vi "OpenMV_SelectLab.vi"(2 "ROI":T1, 3 "image":picture) -> (0 "ROI out":T1, 1 "thresholds":dbl[](array[numeric])=[90.0, 10.0, 20.0, -20.0, 20.0, -20.0])   [LabVIEW 2020]
doc: "This VI pops up a window where the user can select a region of interest."
panel:
  out "Plots":T2
  out "Mouse Down":cluster{"X":i32, "Y":i32}
  out "String":string
  out "Mouse in":bool
  in  "Pen":u32(colorbox)=16774656
  out "overlay":picture caption="Image"
  in  "OK":bool
  out "Display":picture caption="new picture"
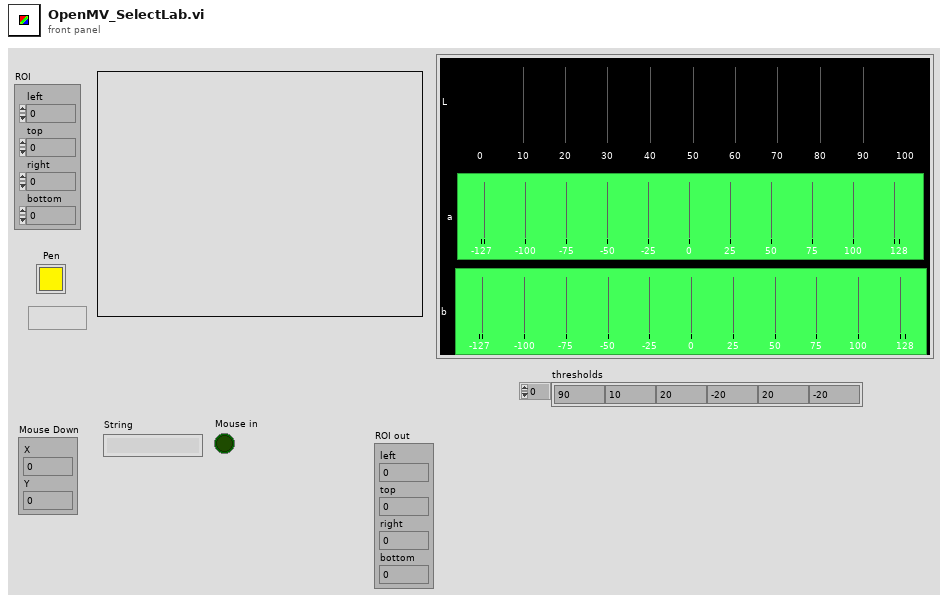
[diagram p1: front panel]
types:
  T1 = cluster{"left":i32, "top":i32, "right":i32, "bottom":i32}
  T2 = cluster{"L":dbl[], "a":cluster{i32, i32, dbl[]}, "b":cluster{i32, i32, dbl[]}}
  T3 = typedef "imagedata.ctl" = cluster{"image type":i32, "image depth":i32, "image":u8[], "mask":u8[], "colors":u32[], "Rectangle":cluster{"left":i16, "top":i16, "right":i16, "bottom":i16}}
  T4 = cluster{"left":i16, "top":i16, "right":i16, "bottom":i16}
  T5 = typedef "LVMouseTypeDef.ctl" = cluster{"Mouse Position":cluster{"X":i32, "Y":i32}, "Mouse Modifiers":cluster{"Button Down":bool, "Shift Mod":bool, "Menu Mod":bool, "Option Mod":bool}}
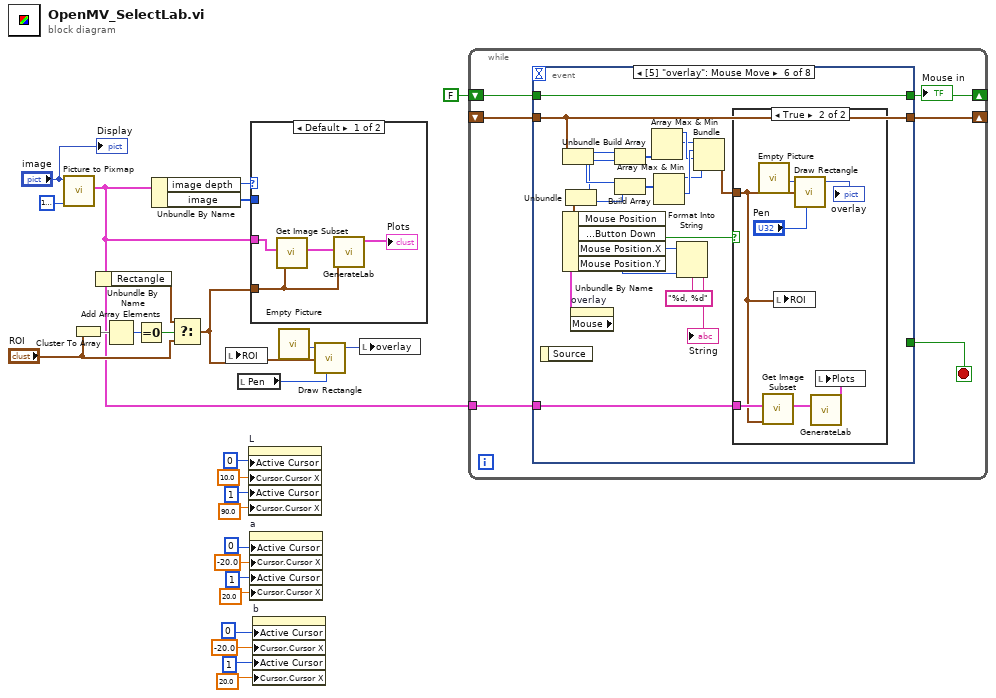
[diagram p0: block diagram]
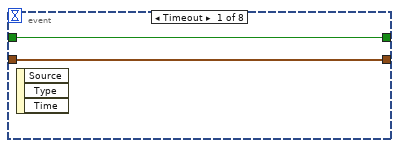
[diagram p3: hidden frame]
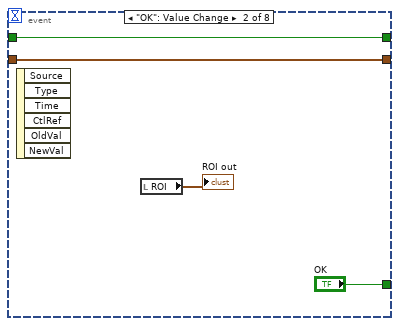
[diagram p4: hidden frame]
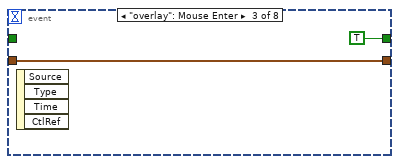
[diagram p5: hidden frame]
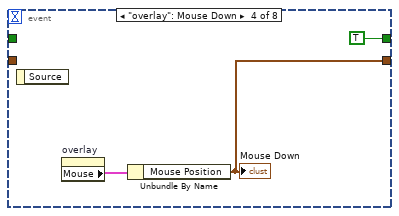
[diagram p6: hidden frame]
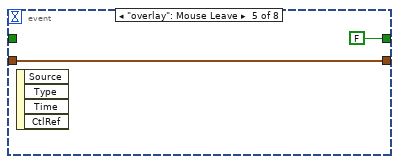
[diagram p7: hidden frame]
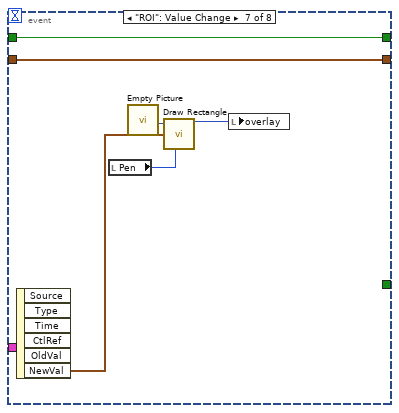
[diagram p9: hidden frame]
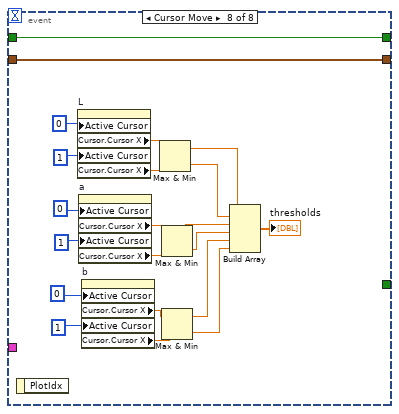
[diagram p10: hidden frame]
diagram:
  n1 = call <vilib>:"Picture to Pixmap.vi"("Background Color"=u32 16777216, "picture"="image") -> ("image data"=w2:T3)  [unwired: 8 in, 1 out]
  n2 = Cluster To Array(cluster="ROI") -> (array=w7:i32[])
  n3 = Unbundle By Name(w2) -> ("Rectangle"=w1:T4)
  n4 = Add Array Elements(numeric array=w7) -> (sum=w6:i32)
  n5 = Equal To 0?(x=w6) -> (x = 0?=w5:bool)
  n6 = Unbundle By Name(w2) -> ("image depth"=w25:i32, "image"=w24:u8[])
  n7 = Select(t=w1, s=w5, f="ROI") -> (s? t:f=w3:T1)
  n8 = local write "ROI"(w3) -> ()
  n9 = local read "Pen"() -> (w8:u32)
  n10 = property on="L" class="WFGraph (strict)"("Active Cursor"=u32 0, "Cursor.Cursor X"=10.0 ("Cursor.Cursor Position:Cursor X"), "Active Cursor"=u32 1, "Cursor.Cursor X"=90.0 ("Cursor.Cursor Position:Cursor X")) -> ()  [unwired: 2 in, 2 out]
  n11 = property on="a" class="WFGraph (strict)"("Active Cursor"=u32 0, "Cursor.Cursor X"=-20.0 ("Cursor.Cursor Position:Cursor X"), "Active Cursor"=u32 1, "Cursor.Cursor X"=20.0 ("Cursor.Cursor Position:Cursor X")) -> ()  [unwired: 2 in, 2 out]
  n12 = case shown="Default" w25 {
    tunnel: w24 -> [_ _]
    tunnel: w2 -> [w30 _]
    tunnel: w3 -> [w28 _]
    frame Default {
      n13 = call <vilib>:"Get Image Subset.vi"("subset rect"=w28, "image data"=w30) -> ("image subset"=w29:T3)  [unwired: 4 in, 1 out]
      n14 = call "GenerateLab.vi"("ROI"=w28, "image data"=w29) -> ("Plots"=→"Plots":T2)  [unwired: 8 in, 1 out]
    }
    frame ..8 {
    }
  }
  n15 = property on="b" class="WFGraph (strict)"("Active Cursor"=u32 0, "Cursor.Cursor X"=-20.0 ("Cursor.Cursor Position:Cursor X"), "Active Cursor"=u32 1, "Cursor.Cursor X"=20.0 ("Cursor.Cursor Position:Cursor X")) -> ()  [unwired: 2 in, 2 out]
  n16 = call "Empty Picture"() -> ("empty picture"=w10:picture)
  n17 = call <vilib>:"Draw Rectangle.vi"("picture"=w10, "rect"=w3, "color(black)"=w8) -> ("new picture"=w9:picture)  [unwired: 6 in]
  n18 = local write "overlay"(w9) -> ()
  n19 = while {
    shift-right: [w36] -> _
    shift-left: FALSE ("Mouse in") -> [w35]
    shift-right: [w34] -> _
    shift-left: _ -> [w33]
    tunnel: w2 -> [w32]
    stop <- w37 stop-if-true
    n20 = event shown="[5] \"overlay\": Mouse Move" {
      selector: _ -> [_ _ _ _ _ _ _ _]
      dyn-events: _ -> [_ _ _ _ _ _ _ _]
      timeout: _ -> [_ _ _ _ _ _ _ _]
      tunnel: [_ "OK" _ _ _ _ _ _] -> w37
      tunnel: [w39 w42 TRUE ("Mouse in") TRUE ("Mouse in") FALSE ("Mouse in") w71 w81 w104] -> w36
      tunnel: w35 -> [w39 w42 _ _ _ w71 w81 w104]
      tunnel: [w38 w41 w44 w46 w49 w59 w80 w105] -> w34
      tunnel: w33 -> [w38 w41 w44 _ w49 w59 w80 w105]
      tunnel: w32 -> [_ _ _ _ _ w51 _ _]
      event Timeout {
        n21 = event-data() -> ()  [unwired: 1 in, 3 out]
      }
      event "OK": Value Change {
        n22 = event-data() -> ()  [unwired: 1 in, 6 out]
        n23 = local read "ROI"() -> (→"ROI out":T1)
      }
      event "overlay": Mouse Enter {
        n24 = event-data() -> ()  [unwired: 1 in, 4 out]
      }
      event "overlay": Mouse Down {
        n25 = event-data() -> ()  [unwired: 1 in, 1 out]
        n26 = property on="overlay" class="Pict"() -> ("Mouse"=w47:T5)  [unwired: 2 in, 2 out]
        n27 = Unbundle By Name(w47) -> ("Mouse Position"=w46:cluster{"X":i32, "Y":i32})
        "Mouse Down" <- w46
      }
      event "overlay": Mouse Leave {
        n28 = event-data() -> ()  [unwired: 1 in, 4 out]
      }
      event "overlay": Mouse Move {
        n29 = event-data() -> ()  [unwired: 1 in, 1 out]
        n30 = Unbundle(w59) -> ("X"=w60:i32, "Y"=w58:i32)
        n31 = property on="overlay" class="Pict"() -> ("Mouse"=w70:T5)  [unwired: 2 in, 2 out]
        n32 = Unbundle By Name(w70) -> ("Mouse Position"=w55:cluster{"X":i32, "Y":i32}, "Mouse Modifiers.Button Down"=w69:bool, "Mouse Position.X"=w67:i32, "Mouse Position.Y"=w66:i32)
        n33 = Unbundle(w55) -> ("X"=w54:i32, "Y"=w53:i32)
        n34 = Build Array(w60, w54) -> (w57:i32[])
        n35 = Build Array(w58, w53) -> (w56:i32[])
        n36 = Array Max & Min(array=w57) -> (max value=w62:i32, min value=w61:i32)  [unwired: 2 out]
        n37 = Array Max & Min(array=w56) -> (max value=w63:i32, min value=w64:i32)  [unwired: 2 out]
        n38 = Format Into String(format string="%d, %d", w67, w66) -> (resulting string=→"String":string)  [unwired: 2 in, 1 out]
        n39 = Bundle(w61, w64, w62, w63) -> (w52:cluster{i32, i32, i32, i32})  [unwired: 1 out]
        n40 = case shown="True" w69 {
          tunnel: w52 -> [_ w72]
          tunnel: w51 -> [_ w75]
          frame False {
          }
          frame True {
            n41 = call "Empty Picture"() -> ("empty picture"=w78:picture)
            n42 = call <vilib>:"Get Image Subset.vi"("subset rect"=w72, "image data"=w75) -> ("image subset"=w74:T3)  [unwired: 4 in, 1 out]
            n43 = local write "ROI"(w72) -> ()
            n44 = call <vilib>:"Draw Rectangle.vi"("picture"=w78, "rect"=w72, "color(black)"="Pen") -> ("new picture"=→"overlay":picture)  [unwired: 6 in]
            n45 = call "GenerateLab.vi"("image data"=w74) -> ("Plots"=w73:T2)  [unwired: 9 in, 1 out]
            n46 = local write "Plots"(w73) -> ()
          }
        }
      }
      event "ROI": Value Change {
        n47 = event-data() -> ("NewVal"=w79:T1)  [unwired: 1 in, 5 out]
        n48 = local read "Pen"() -> (w82:u32)
        n49 = call "Empty Picture"() -> ("empty picture"=w84:picture)
        n50 = call <vilib>:"Draw Rectangle.vi"("picture"=w84, "rect"=w79, "color(black)"=w82) -> ("new picture"=w83:picture)  [unwired: 6 in]
        n51 = local write "overlay"(w83) -> ()
      }
      event "Plots.L", "Plots.a", "Plots.b": Cursor Move {
        n52 = event-data() -> ()  [unwired: 1 in, 1 out]
        n53 = property on="L" class="WFGraph (strict)"("Active Cursor"=u32 0, "Active Cursor"=u32 1) -> ("Cursor.Cursor X"=w95:dbl, "Cursor.Cursor X"=w96:dbl)  [unwired: 2 in, 2 out]
        n54 = property on="a" class="WFGraph (strict)"("Active Cursor"=u32 0, "Active Cursor"=u32 1) -> ("Cursor.Cursor X"=w92:dbl, "Cursor.Cursor X"=w91:dbl)  [unwired: 2 in, 2 out]
        n55 = property on="b" class="WFGraph (strict)"("Active Cursor"=u32 0, "Active Cursor"=u32 1) -> ("Cursor.Cursor X"=w88:dbl, "Cursor.Cursor X"=w87:dbl)  [unwired: 2 in, 2 out]
        n56 = Max & Min(x=w95, y=w96) -> (max(x,y)=w94:dbl, min(x,y)=w93:dbl)
        n57 = Max & Min(x=w92, y=w91) -> (max(x,y)=w90:dbl, min(x,y)=w89:dbl)
        n58 = Max & Min(x=w88, y=w87) -> (max(x,y)=w86:dbl, min(x,y)=w85:dbl)
        n59 = Build Array(w94, w93, w90, w89, w86, w85) -> (→"thresholds":dbl[])
      }
    }
    "Mouse in" <- w36
  }
  "Display" <- "image"
